vi "Interface-RS232.vi"(8 "stop":bool, 10 "COM Port":string="COM3", 11 "Sensor type":string="ild1402") -> (3 "ScaledData":dbl[](graph))   [LabVIEW 2015, in "MEDAQLib.lvlib"]
uses:
  Documents/MEDAQLib-4.11.1.31486/Samples/LabView/MEDAQLib/MEDAQLib.lvlib
panel:
  in  "stop 2":bool
  out "ScaledData 2":dbl[](graph)
  out "subarray":dbl[](array[numeric])
  out "Last error text":string
  in  "Block size":i32=200
  # "1. Preparations\nPlease use Sensor tool to find sensor connected to your PC and get its interface/communication parameters."
  # "2. Inform MEDAQLib about sensor type and interface parameters.\nFor possible sensor type names see MEDAQLib.h or CreateSensorInstByName documentation in MEDAQLib.pdf\nCOM Port = Portname\nPlease note: this example expects to access the sensor with its default baudrate. You may need to insert another SetParameterInt VI to tell MEDAQLib about a changed baudrate."
  # "3. Start LabView execution"
  # "4.For stop please do not use LabView red stop button on toolbar, but the red STOP button below to be able to inform MEDAQLib about release of sensor instance information."
  # "Number of samples\nper transfered data block"
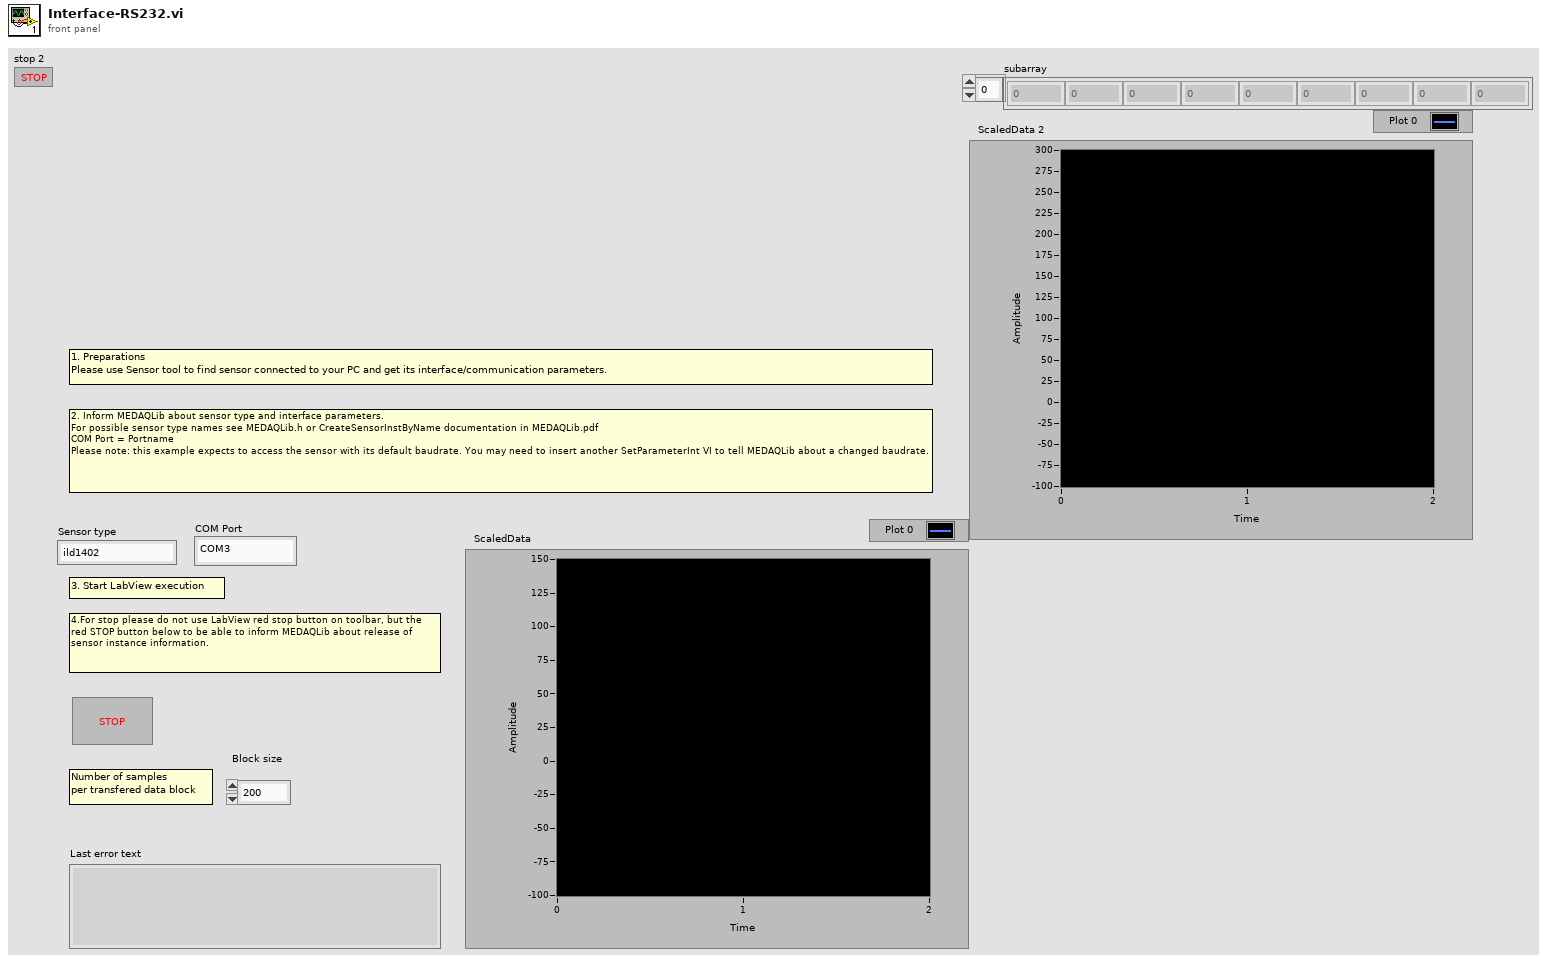
[diagram p1: front panel]
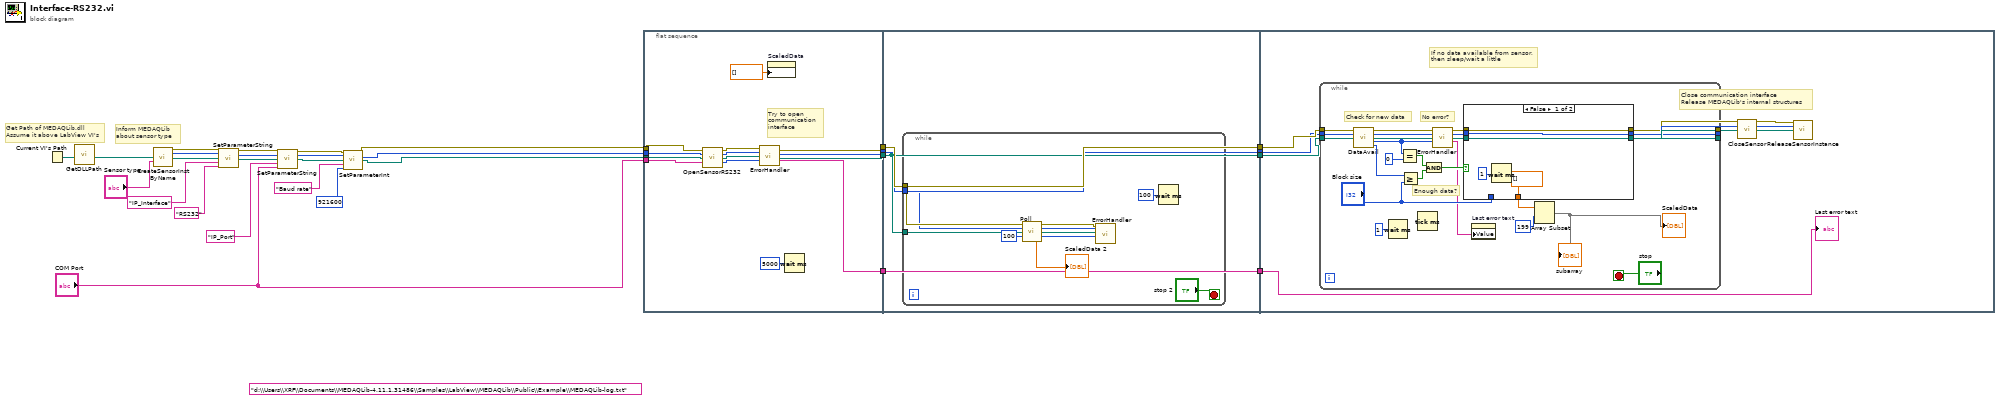
[diagram p0: block diagram]
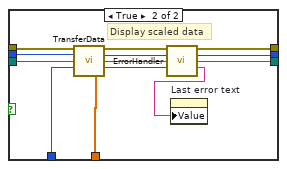
[diagram p2: hidden frame]
diagram:
  (unwired) "d:\\Users\\XRF\\Documents\\MEDAQLib-4.11.1.31486\\Samples\\LabView\\MEDAQLib\\Public\\Example\\MEDAQLib-log.txt" ("paramValue")
  # "Inform MEDAQLib\nabout sensor type"
  # "Get Path of MEDAQLib.dll\nAssume it above LabView VI's"
  n1 = Current VI's Path() -> (path=w27:path)
  n2 = call "GetDLLPath.vi"("VI-Path"=w27) -> ("DLL-Path"=w28:path)  [unwired: 10 out]
  n3 = call "CreateSensorInstByName.vi"("DLL-Path"=w28, "sensor"="Sensor type") -> ("Fehler (Ausgang)"=w17:errorcluster, "instanceHandle"=w14:u32, "DLL-Path"=w8:path)  [unwired: 1 in, 10 out]
  n4 = call "SetParameterString.vi"("Fehler (Eingang, kein Fehler)"=w17, "instanceHandle"=w14, "DLL-Path"=w8, "paramName"="IP_Interface", "paramValue"="RS232") -> ("Fehler (Ausgang)"=w18:errorcluster, "instanceHandle"=w13:u32, "DLL-Path"=w9:path)  [unwired: 7 in, 1 out]
  n5 = call "SetParameterString.vi"("Fehler (Eingang, kein Fehler)"=w18, "instanceHandle"=w13, "DLL-Path"=w9, "paramName"="IP_Port", "paramValue"="COM Port") -> ("Fehler (Ausgang)"=w16:errorcluster, "instanceHandle"=w12:u32, "DLL-Path"=w10:path)  [unwired: 7 in, 1 out]
  n6 = call "SetParameterInt.vi"("Fehler (Eingang, kein Fehler)"=w16, "instanceHandle"=w12, "DLL-Path"=w10, "paramName"="Baud rate", "paramValue"=921600) -> ("Fehler (Ausgang)"=w15:errorcluster, "instanceHandle"=w7:u32, "DLL-Path"=w11:path)  [unwired: 7 in, 1 out]
  n7 = flat-sequence {
    tunnel: w15 -> [w35]
    tunnel: w11 -> [w34]
    tunnel: w7 -> [w33]
    tunnel: "COM Port" -> [w32]
    tunnel: [w43] -> w26
    tunnel: [w42] -> w24
    tunnel: [w41] -> w22
    tunnel: [w40] -> w20
    tunnel: w26 -> [w46]
    tunnel: [w46] -> w25
    tunnel: w24 -> [w45]
    tunnel: [w45] -> w23
    tunnel: w22 -> [w44]
    tunnel: [w44] -> w21
    tunnel: w20 -> [w47]
    tunnel: [w47] -> w19
    tunnel: w25 -> [w62]
    tunnel: w23 -> [w61]
    tunnel: w21 -> [w60]
    tunnel: w19 -> [w59]
    frame #0 {
      # "Try to open\ncommunication\ninterface"
      n8 = call "OpenSensorRS232.vi"("Fehler (Eingang, kein Fehler)"=w35, "instanceHandle"=w33, "DLL-Path"=w34, "port"=w32) -> ("Fehler (Ausgang)"=w39:errorcluster, "instanceHandle"=w38:u32, "DLL-Path"=w37:path, "ERR_CODE"=w36:i32)  [unwired: 8 in]
      n9 = call "ErrorHandler.vi"("Fehler (Eingang, kein Fehler)"=w39, "instanceHandle"=w38, "DLL-Path"=w37, "ERR_CODE"=w36) -> ("Fehler (Ausgang)"=w43:errorcluster, "instanceHandle"=w42:u32, "DLL-Path"=w41:path, "errText"=w40:string)  [unwired: 8 out]
      n10 = property on="ScaledData" class="WFChart (strict)"("History Data"=dbl[] []) -> ()  [unwired: 2 in, 2 out]
      n11 = Wait (ms)(milliseconds to wait=u32 5000 ("Zu wartende ms")) -> ()  [unwired: 1 out]
    }
    frame #1 {
      n12 = while {
        tunnel: w46 -> [w58]
        tunnel: w45 -> [w57]
        tunnel: w44 -> [w56]
        stop <- "stop 2" stop-if-true
        n13 = call "Poll.vi"("Fehler (Eingang, kein Fehler)"=w58, "instanceHandle"=w57, "DLL-Path"=w56, "maxValues"=100) -> ("Fehler (Ausgang)"=w53:errorcluster, "instanceHandle"=w52:u32, "DLL-Path"=w51:path, "ERR_CODE"=w50:i32, "scaledData"=→"ScaledData 2":dbl[])  [unwired: 6 in, 1 out]
        n14 = call "ErrorHandler.vi"("Fehler (Eingang, kein Fehler)"=w53, "instanceHandle"=w52, "DLL-Path"=w51, "ERR_CODE"=w50) -> ()  [unwired: 12 out]
        n15 = Wait (ms)(milliseconds to wait=u32 100 ("Zu wartende ms")) -> ()  [unwired: 1 out]
      }
    }
    frame #2 {
      # "If no data available from sensor,\nthen sleep/wait a little"
      # "Close communication interface\nRelease MEDAQLib's internal structures"
      n16 = while {
        tunnel: w62 -> [w93]
        tunnel: w61 -> [w92]
        tunnel: w60 -> [w91]
        tunnel: [w86] -> w63
        tunnel: [w85] -> w64
        tunnel: [w84] -> w65
        stop <- "stop" stop-if-true
        # "Enough data?"
        # "No error?"
        # "Check for new data"
        n17 = call "DataAvail.vi"("Fehler (Eingang, kein Fehler)"=w93, "instanceHandle"=w92, "DLL-Path"=w91) -> ("Fehler (Ausgang)"=w80:errorcluster, "instanceHandle"=w78:u32, "DLL-Path"=w76:path, "ERR_CODE"=w74:i32, "avail"=w90:i32)  [unwired: 8 out]
        n18 = Wait (ms)(milliseconds to wait=u32 1 ("Zu wartende ms")) -> ()  [unwired: 1 out]
        n19 = Equal?(x=w74, y=0 ("x")) -> (x = y?=w87:bool)
        n20 = Greater Or Equal?(x=w90, y="Block size") -> (x >= y?=w83:bool)
        n21 = Tick Count (ms)() -> ()  [unwired: 1 out]
        n22 = And(x=w87, y=w83) -> (x .and. y?=w88:bool)
        n23 = call "ErrorHandler.vi"("Fehler (Eingang, kein Fehler)"=w80, "instanceHandle"=w78, "DLL-Path"=w76, "ERR_CODE"=w74) -> ("Fehler (Ausgang)"=w79:errorcluster, "instanceHandle"=w77:u32, "DLL-Path"=w75:path, "errText"=w73:string)  [unwired: 8 out]
        n24 = case shown="False" w88 {
          tunnel: w79 -> [w98 w110]
          tunnel: w77 -> [w97 w111]
          tunnel: w75 -> [w96 w109]
          tunnel: [w98 w106] -> w86
          tunnel: [w97 w104] -> w85
          tunnel: [w96 w102] -> w84
          tunnel: "Block size" -> [_ w108]
          tunnel: [dbl[] [] ("scaledData") w99] -> w70
          frame False {
            n25 = Wait (ms)(milliseconds to wait=u32 1 ("Zu wartende ms")) -> ()  [unwired: 1 out]
          }
          frame True {
            # "Display scaled data"
            n26 = call "TransferData.vi"("Fehler (Eingang, kein Fehler)"=w110, "instanceHandle"=w111, "DLL-Path"=w109, "maxValues"=w108) -> ("Fehler (Ausgang)"=w107:errorcluster, "instanceHandle"=w105:u32, "DLL-Path"=w103:path, "ERR_CODE"=w101:i32, "scaledData"=w99:dbl[])  [unwired: 7 out]
            n27 = call "ErrorHandler.vi"("Fehler (Eingang, kein Fehler)"=w107, "instanceHandle"=w105, "DLL-Path"=w103, "ERR_CODE"=w101) -> ("Fehler (Ausgang)"=w106:errorcluster, "instanceHandle"=w104:u32, "DLL-Path"=w102:path, "errText"=w100:string)  [unwired: 8 out]
            n28 = property on="Last error text" class="Str"("Value"=w100) -> ()  [unwired: 2 in, 2 out]
          }
        }
        n29 = property on="Last error text" class="Str"("Value"=w73) -> ()  [unwired: 2 in, 2 out]
        n30 = Array Subset(array=w70, index=199) -> (→"subarray" →"ScaledData":dbl[])  [unwired: 1 in]
      }
      n31 = call "CloseSensor.vi"("Fehler (Eingang, kein Fehler)"=w63, "instanceHandle"=w64, "DLL-Path"=w65) -> ("Fehler (Ausgang)"=w66:errorcluster, "instanceHandle"=w67:u32, "DLL-Path"=w68:path)  [unwired: 10 out]
      n32 = call "ReleaseSensorInstance.vi"("Fehler (Eingang, kein Fehler)"=w66, "instanceHandle"=w67, "DLL-Path"=w68) -> ()  [unwired: 13 out]
      "Last error text" <- w59
    }
  }
